vi "Configure View Model.vi"(8 "error in (no error)":errorcluster, 10 "List Box View Model":refnum<class "Process Tree View Model.lvclass">, 11 "List Box View In":refnum<class "Process Tree View.lvclass">) -> (0 "error out":errorcluster, 3 "List Box View Out":refnum<class "Process Tree View.lvclass">)   [LabVIEW 2020, in "Process Tree View.lvclass"]
uses:
  Process Tree View.lvclass
  Process Tree View.lvclass/Process Tree View.ctl
  Process Tree View Model/Process Tree View Model.lvclass
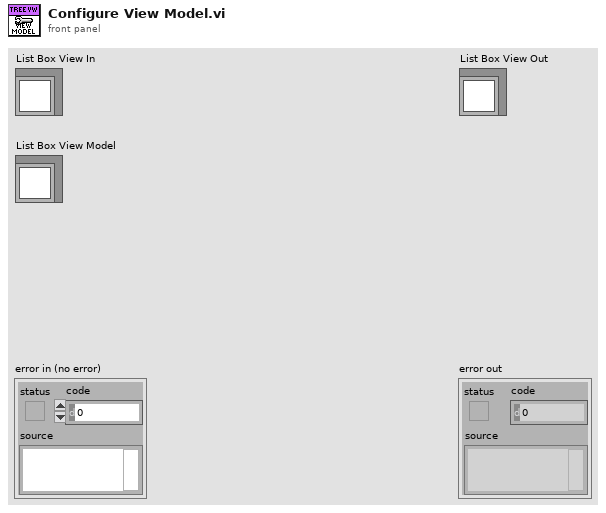
[diagram p1: front panel]
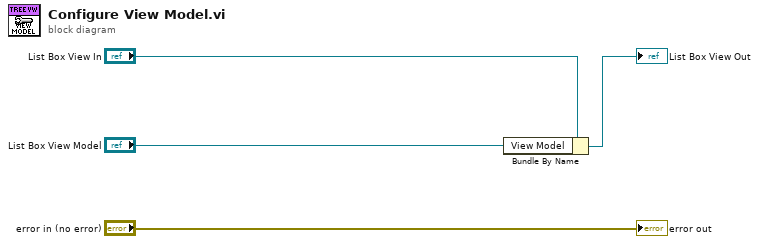
[diagram p0: block diagram]
diagram:
  n1 = Bundle By Name(cluster="List Box View In", "View Model"="List Box View Model") -> (→"List Box View Out":refnum<class "Process Tree View.lvclass">)
  "error out" <- "error in (no error)"
